vi "Closedown.vi"(8 "error In":errorcluster, 10 "DeviceKey In":string, 11 "CmdLib In":refnum<k24>) -> (0 "error out":errorcluster)   [LabVIEW 2020]
uses:
  C:/GEECS/Developers Version/builds/Device builds/Picomotor8742dotNet/CmdLib.dll
  CmdLib.dll
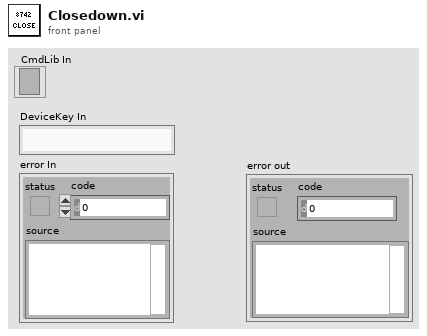
[diagram p1: front panel]
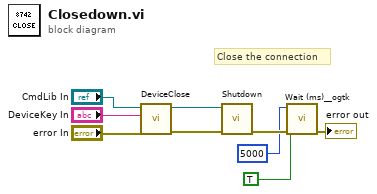
[diagram p0: block diagram]
diagram:
  # "Close the connection"
  n1 = call "DeviceClose.vi"("error in (no error)"="error In", "DeviceKey In"="DeviceKey In", "CmdLib In"="CmdLib In") -> ("error out"=w9:errorcluster, "CmdLib Out"=w8:refnum<k24>)  [unwired: 2 in, 1 out]
  n2 = call "Shutdown.vi"("error in (no error)"=w9, "CmdLib In"=w8) -> ("error out"=w4:errorcluster)  [unwired: 4 in, 1 out]
  n3 = call "Wait (ms)__ogtk.vi"("error in (no error)"=w4, "Wait on Error (FALSE)"=TRUE, "milliseconds to wait"=u32 5000) -> ("error out"=→"error out":errorcluster)  [unwired: 7 in, 1 out]
